vi "Is Bus Monitor.vi"(8 "error in (no error)":errorcluster, 11 "1553 SubComponent":refnum<class "1553 SubComponent.lvclass">) -> (0 "error out":errorcluster)   [LabVIEW 2016, in "BCI-1553 API.lvlib" / "1553 Component.lvclass"]
uses:
  1553 Component.lvclass
  Bus Monitor/Bus Monitor.lvclass
  1553 SubComponent/1553 SubComponent.lvclass
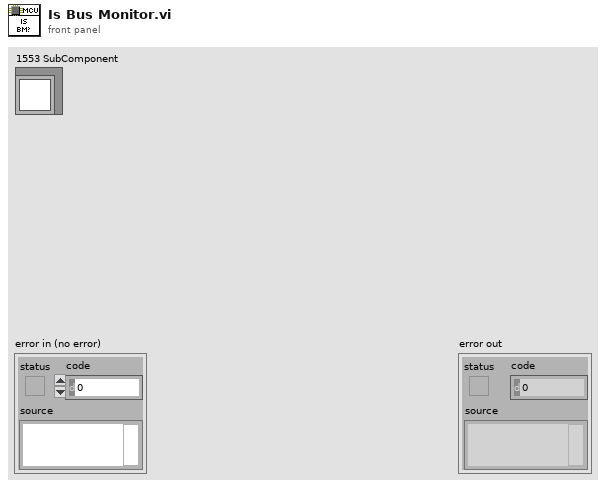
[diagram p1: front panel]
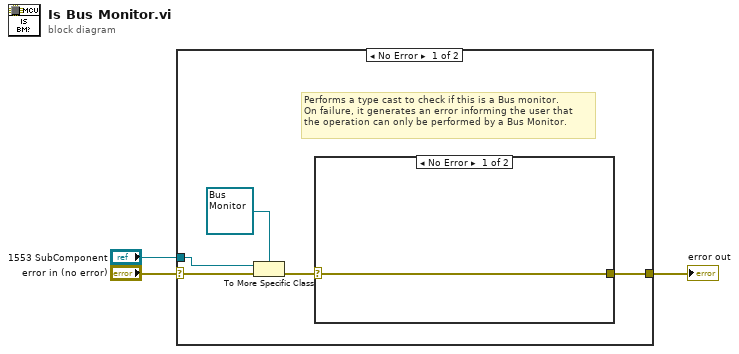
[diagram p0: block diagram]
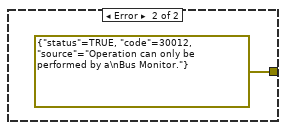
[diagram p2: hidden frame]
diagram:
  n1 = case shown="No Error" "error in (no error)" {
    selector: "error in (no error)" -> [w6 w11]
    tunnel: [w8 w11] -> w1
    tunnel: "1553 SubComponent" -> [w7 _]
    frame No Error {
      # "Performs a type cast to check if this is a Bus monitor.\nOn failure, it generates an error informing the user that\nthe operation can only be performed by a Bus Monitor."
      n2 = To More Specific Class(target class=refnum<class "Bus Monitor.lvclass"> refnum ("BCI-1553 API.lvlib:Bus Monitor.lvclass"), reference=w7, error in=w6) -> (error out=w5:errorcluster)  [unwired: 1 out]
      n3 = case shown="No Error" w5 {
        selector: w5 -> [w9 _]
        tunnel: [w9 errorcluster {"status"=TRUE, "code"=30012, "source"="Operation can only be performed by a\nBus Monitor."} ("error IO")] -> w8
        frame No Error {
        }
        frame Error {
        }
      }
    }
    frame Error {
    }
  }
  "error out" <- w1
